vi "CoriolisEner.vi"() -> ()   [LabVIEW 2021]
panel:
  out "Tab Control":T1(tab)
  in  "Tab Control 3":enum32{"Comunicación", "Medidores"}(tab)
  in  "Paridad":string(combo)="Even"
  in  "Baudrate":string(combo)="9600"
  in  "COM Port":refnum<visa-resource-name>
  in  "Multicolumn Listbox":i32(listbox)
  in  "Tab Control 2":T2(tab)
  out "Corriente I3":dbl(knob) scale=0.0..900.0
  out "Corriente I2":dbl(knob) scale=0.0..900.0
  out "Corriente I1":dbl(knob) scale=0.0..900.0
  out "Voltaje L13":dbl(knob) scale=0.0..300.0
  out "Voltaje L21":dbl(knob) scale=0.0..300.0
  out "Voltaje L12":dbl(knob) scale=0.0..300.0
  out "Tabla VIF":string[][](table)
  out "Voltaje L-L":cluster{timestamp[], dbl[]}[](graph)
  out "FP":dbl(knob) scale=-1.0..1.0
  out "Hz":dbl(knob) scale=45.0..65.0
  out "Corriente":cluster{timestamp[], dbl[]}[](graph)
  out "KVAR":cluster{timestamp[], dbl[]}[](graph)
  out "FP":cluster{timestamp[], dbl[]}[](graph)
  out "KWT":cluster{timestamp[], dbl[]}(graph)
  out "Potencia":string[][](table)
  in  "Text Ring":u16(ring)
  in  "current time 2":timestamp format="%<%d/%m/%Y>T"
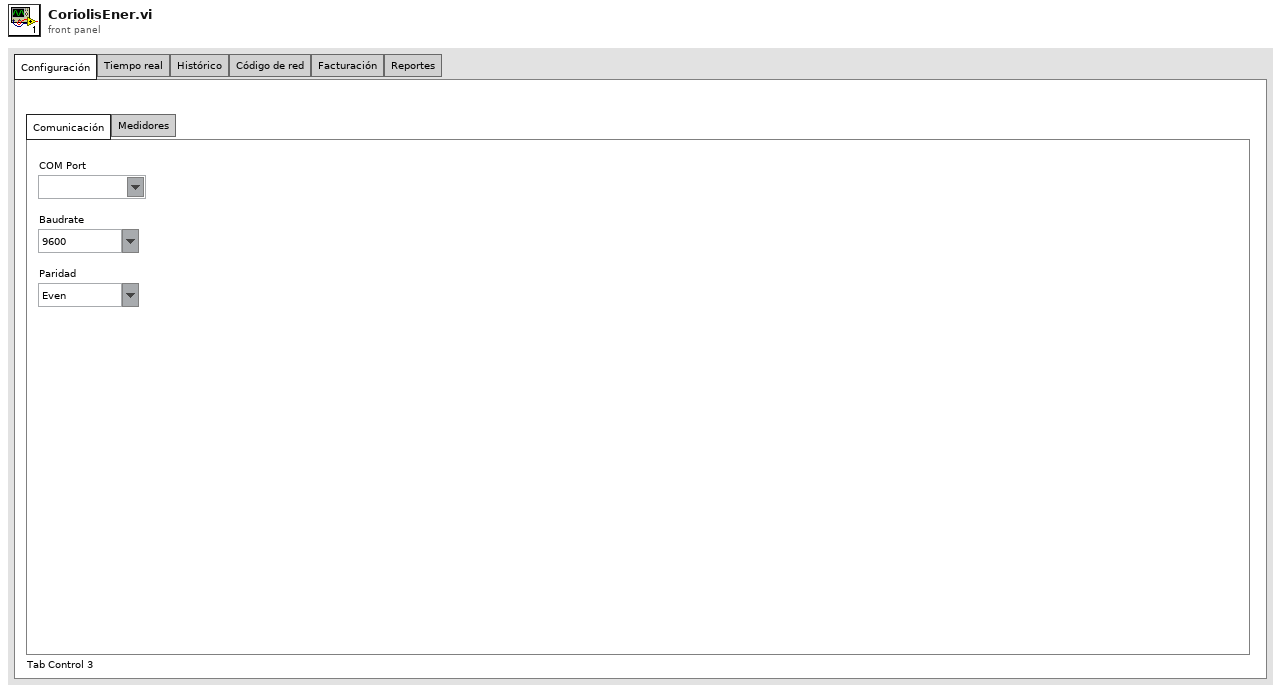
[diagram p1: front panel]
types:
  T1 = enum32{"Configuración", "Tiempo real", "Histórico", "Código de red", "Facturación", "Reportes"}
  T2 = enum32{"VIF", "Potencia", "Energía", "Armónicos"}
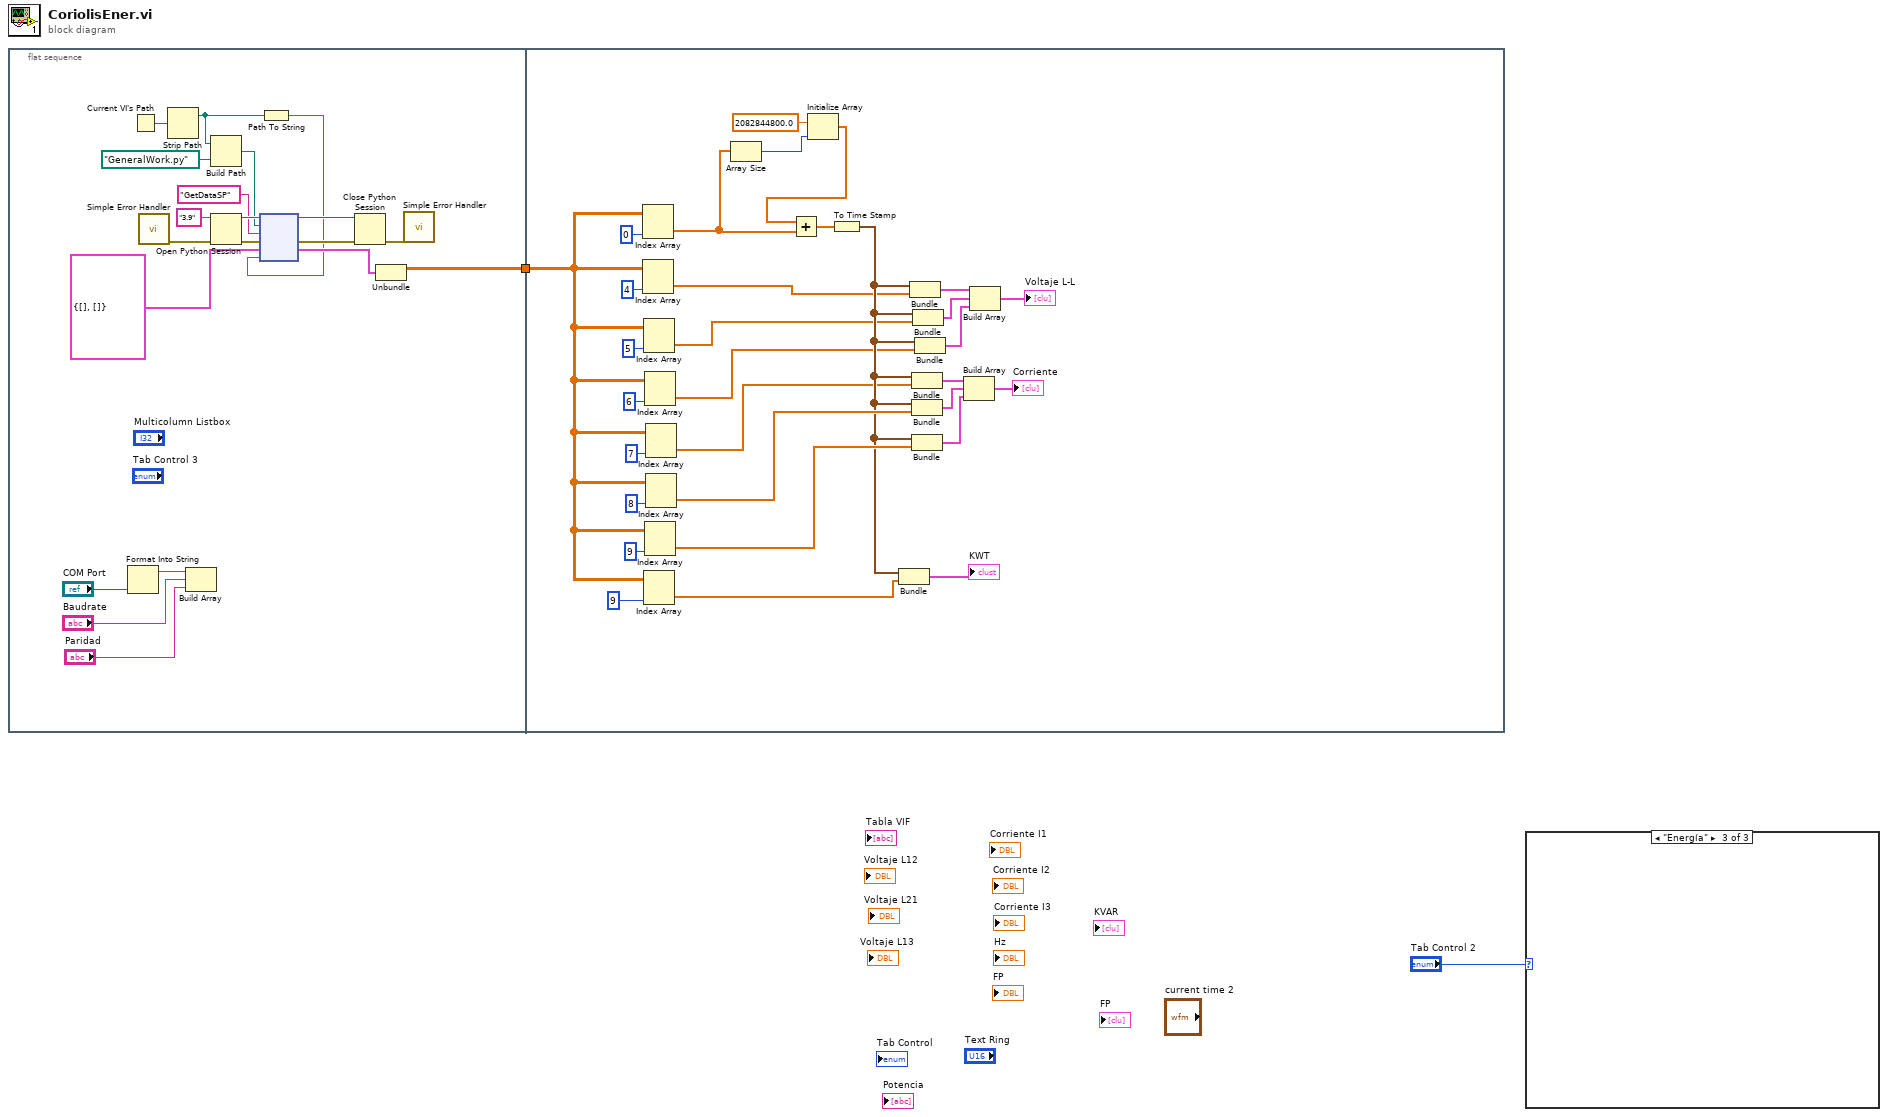
[diagram p0: block diagram]
diagram:
  n1 = flat-sequence {
    tunnel: [w7] -> w1
    tunnel: w1 -> [w24]
    frame #0 {
      n2 = Format Into String("COM Port") -> (resulting string=w6:string)  [unwired: 3 in, 1 out]
      n3 = Current VI's Path() -> (path=w15:path)
      n4 = call <vilib>:"Simple Error Handler.vi"() -> ("error out"=w9:errorcluster)  [unwired: 5 in, 4 out]
      n5 = Strip Path(path=w15) -> (stripped path=w14:path)  [unwired: 1 out]
      n6 = Build Array(w6, "Baudrate", "Paridad") -> ()  [unwired: 1 out]
      n7 = Build Path(base path=w14, name or relative path=path "GeneralWork.py" ("python path")) -> (appended path=w17:path)
      n8 = Open Python Session(python version="3.9" ("Python version"), 3:w9) -> (session out=w20:refnum<k35>, error out=w19:errorcluster)  [unwired: 1 in]
      n9 = Path To String(path=w14) -> (string=w11:string)
      n10 = node(w20, w17, "GetDataSP" ("function name in"), w19, cluster{dbl[][], i32[][]} {[], []}, w11) -> (w22:refnum<k35>, w21:errorcluster, w12:cluster{dbl[][], i32[][]})  [unwired: 1 in, 2 out]
      n11 = Close Python Session(session in=w22, error in=w21) -> (11:w10:errorcluster)
      n12 = Unbundle(w12) -> (w7:dbl[][])  [unwired: 1 out]
      n13 = call <vilib>:"Simple Error Handler.vi"("error in (no error)"=w10) -> ()  [unwired: 4 in, 5 out]
    }
    frame #1 {
      n14 = Index Array(array=w24, index (col)=0 ("disabled index (col)")) -> (element=w34:dbl[])  [unwired: 1 in]
      n15 = Index Array(array=w24, index (col)=4 ("disabled index (col)")) -> (element=w39:dbl[])  [unwired: 1 in]
      n16 = Index Array(array=w24, index (col)=5 ("disabled index (col)")) -> (element=w43:dbl[])  [unwired: 1 in]
      n17 = Index Array(array=w24, index (col)=9 ("disabled index (col)")) -> (element=w40:dbl[])  [unwired: 1 in]
      n18 = Index Array(array=w24, index (col)=6 ("disabled index (col)")) -> (element=w46:dbl[])  [unwired: 1 in]
      n19 = Index Array(array=w24, index (col)=9 ("disabled index (col)")) -> (element=w52:dbl[])  [unwired: 1 in]
      n20 = Index Array(array=w24, index (col)=7 ("disabled index (col)")) -> (element=w33:dbl[])  [unwired: 1 in]
      n21 = Index Array(array=w24, index (col)=8 ("disabled index (col)")) -> (element=w51:dbl[])  [unwired: 1 in]
      n22 = Array Size(array=w34) -> (size(s)=w35:i32)
      n23 = Initialize Array(2082844800.0 ("element"), w35) -> (w36:dbl[])
      n24 = Add(x=w36, y=w34) -> (x+y=w37:dbl[])
      n25 = To Time Stamp(1:w37) -> (0:w50:timestamp[])
      n26 = Bundle(w50, w40) -> (→"KWT":cluster{timestamp[], dbl[]})  [unwired: 1 in]
      n27 = Bundle(w50, w39) -> (w42:cluster{timestamp[], dbl[]})  [unwired: 1 in]
      n28 = Bundle(w50, w33) -> (w48:cluster{timestamp[], dbl[]})  [unwired: 1 in]
      n29 = Bundle(w50, w51) -> (w49:cluster{timestamp[], dbl[]})  [unwired: 1 in]
      n30 = Bundle(w50, w52) -> (w53:cluster{timestamp[], dbl[]})  [unwired: 1 in]
      n31 = Bundle(w50, w43) -> (w44:cluster{timestamp[], dbl[]})  [unwired: 1 in]
      n32 = Bundle(w50, w46) -> (w47:cluster{timestamp[], dbl[]})  [unwired: 1 in]
      n33 = Build Array(w48, w49, w53) -> (→"Corriente":cluster{timestamp[], dbl[]}[])
      n34 = Build Array(w42, w44, w47) -> (→"Voltaje L-L":cluster{timestamp[], dbl[]}[])
    }
  }
  n35 = case shown="\"Energía\"" "Tab Control 2" {
    frame "VIF", Default {
    }
    frame "Potencia" {
    }
    frame "Energía" {
    }
  }
